vi "Subscribe Event.vi"(8 "error in (no error)":errorcluster, 11 "reference in":T1) -> (0 "error out":errorcluster, 3 "reference out":T1)   [LabVIEW 2018]
uses:
  EventClient_ObjectReference.ctl
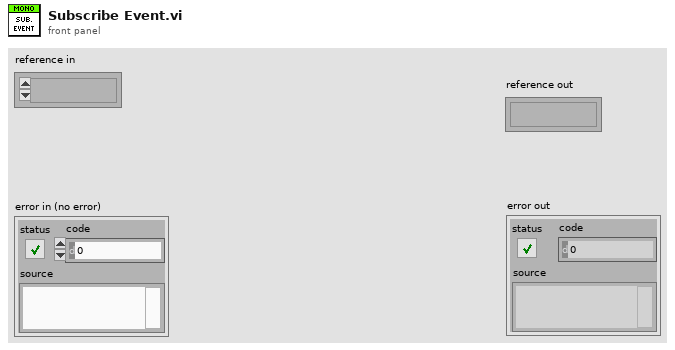
[diagram p1: front panel]
types:
  T1 = typedef "EventClient_ObjectReference.ctl" = refnum<k1>
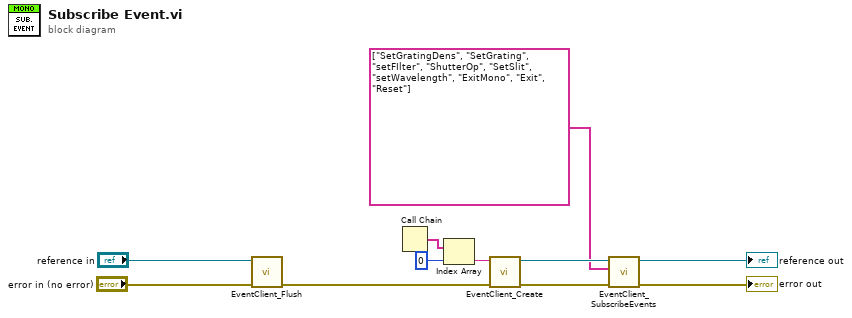
[diagram p0: block diagram]
diagram:
  n1 = call "EventClient_Flush.vi"("error in (no error)"="error in (no error)", "reference"="reference in") -> ("error out"=w1:errorcluster)  [unwired: 8 in, 1 out]
  n2 = Call Chain() -> (call chain=w11:string[])
  n3 = Index Array(array=w11, index=0) -> (element=w9:string)
  n4 = call "EventClient_Create.vi"("error in (no error)"=w1, "Instance Name"=w9) -> ("error out"=w8:errorcluster, "reference"=w7:T1)  [unwired: 8 in]
  n5 = call "EventClient_SubscribeEvents.vi"("error in (no error)"=w8, "Events"=string[] ["SetGratingDens", "SetGrating", "setFIlter", "ShutterOp", "SetSlit", "setWavelength", "ExitMono", "Exit", "Reset"], "reference"=w7) -> ("error out"=→"error out":errorcluster, "reference out"=→"reference out":T1)  [unwired: 7 in]
